vi "gauss on P&D.vi"(3 "error in (no error)":errorcluster, 4 "Coordinates":i32[](array[numeric]), 5 "click event":i32, 6 "gauss fit":bool) -> (0 "error out":errorcluster, 1 "fitted \ncoordinates":i32[](array[numeric]), 2 "Fit successful":bool)   [LabVIEW 2009]
uses:
  <vilib>/vision/NI_Vision_Development_Module.lvlib
panel:
  out "selection":T1(plugin-control)
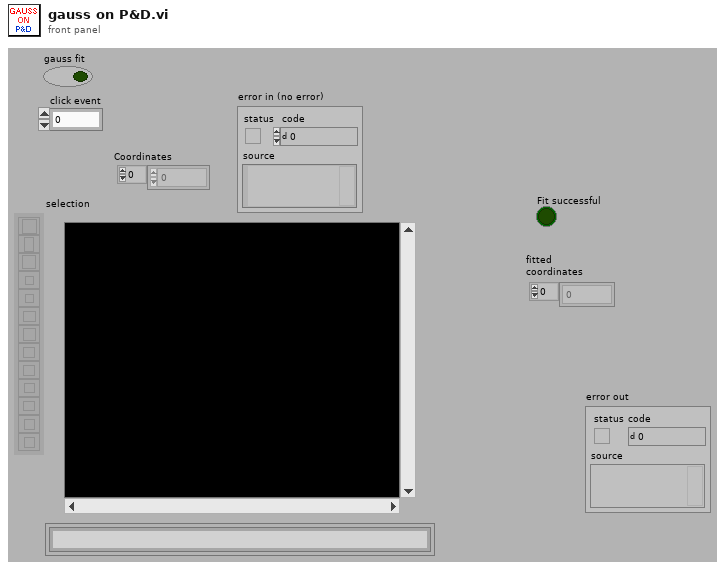
[diagram p1: front panel]
types:
  T1 = typedef "IMAQ Image.ctl" = refnum<image>
  T2 = typedef "DAQLinescanVisualization.ctt" = cluster{"Threshold":u32, "Trace Window #":u32, "IMAQ Trace":T1, "Retrace Window #":u32, "IMAQ Retrace":T1}
  T3 = typedef "Image Type" = u32
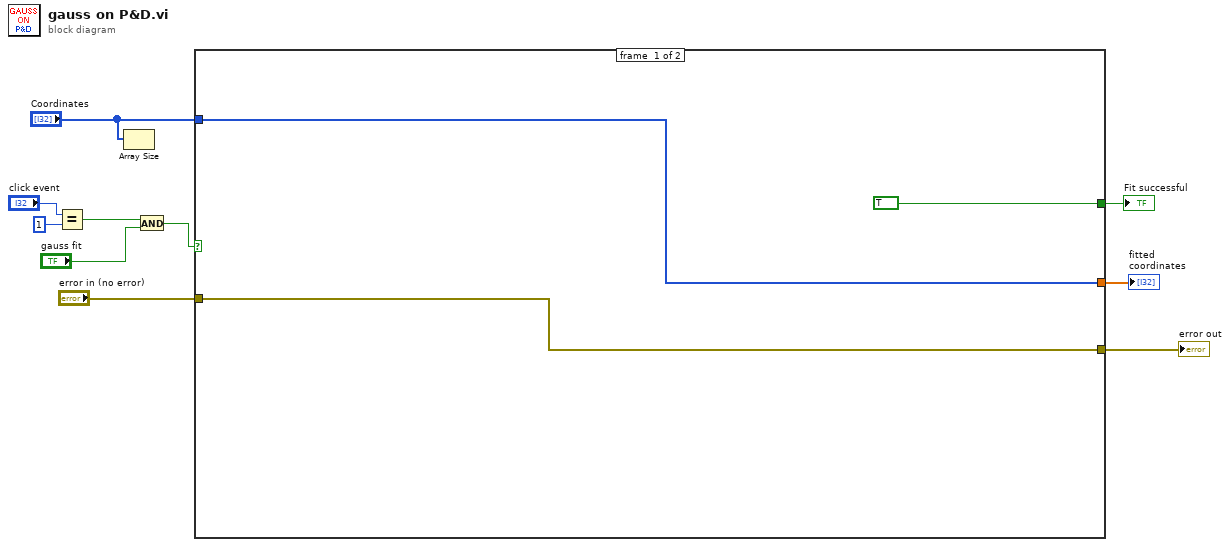
[diagram p0: block diagram]
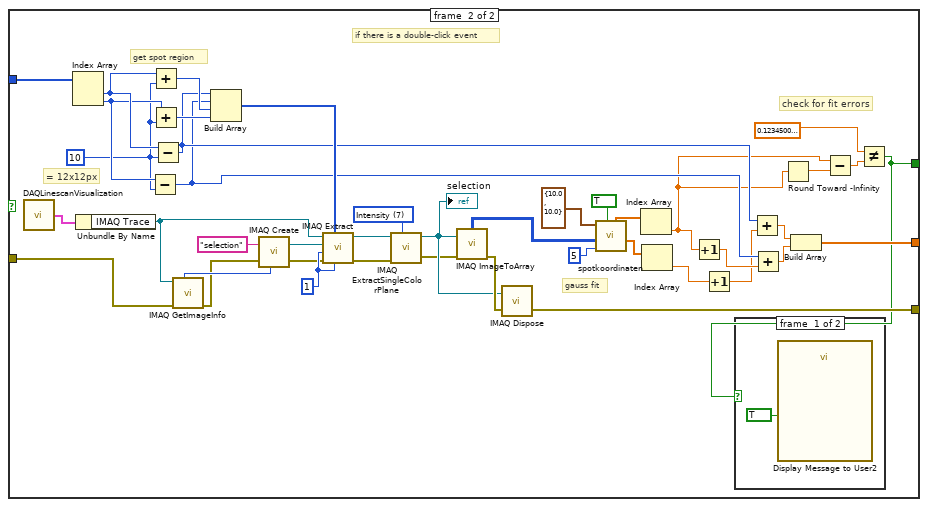
[diagram p2: hidden frame]
diagram:
  n1 = Equal?(x="click event", y=1) -> (x = y?=w2:bool)
  n2 = Array Size(array="Coordinates") -> ()  [unwired: 1 out]
  n3 = And(x=w2, y="gauss fit") -> (x .and. y?=w1:bool)
  n4 = case shown="True" w1 {
    tunnel: "Coordinates" -> [w12 w55]
    tunnel: "error in (no error)" -> [w13 w33]
    tunnel: [w13 w30] -> w8
    tunnel: [w12 w38] -> w7
    tunnel: [TRUE w29] -> w6
    frame #0 {
    }
    frame #1 {
      w24 = 7 items=["Red", "Green", "Blue", "Hue", "Saturation", "Luminance", "Value", "Intensity"] ("Color Plane")
      w51 = 10
      w52 = 1 ("X Step Size")
      # "check for fit errors"
      # "gauss fit"
      # "= 12x12px"
      # "get spot region"
      # "if there is a double-click event"
      n5 = call "DAQLinescanVisualization.vi"() -> ("Visualization (output)"=w27:T2)  [unwired: 2 in]
      n6 = Index Array(array=w55) -> (element #1=w54:i32, element #2=w53:i32)  [unwired: 2 in]
      n7 = Unbundle By Name(w27) -> ("IMAQ Trace"=w35:T1)
      n8 = Subtract(x=w53, y=w51) -> (x-y=w18:i32)
      n9 = Add(x=w54, y=w51) -> (x+y=w21:i32)
      n10 = Add(x=w53, y=w51) -> (x+y=w20:i32)
      n11 = Subtract(x=w54, y=w51) -> (x-y=w19:i32)
      n12 = call "IMAQ GetImageInfo"("error in (no error)"=w33, "Image"=w35) -> ("error out"=w32:errorcluster, "Image Type"=w34:T3)  [unwired: 2 in, 6 out]
      n13 = Build Array(w19, w18, w21, w20) -> (w50:i32[])
      n14 = call "IMAQ Create"("Image Name"="selection", "Image Type"=w34, "error in (no error)"=w32) -> ("New Image"=w42:T1, "error out"=w41:errorcluster)  [unwired: 2 in]
      n15 = call "IMAQ Extract"("Y Step Size"=w52, "Optional Rectangle"=w50, "error in (no error)"=w41, "X Step Size"=w52, "Image Dst"=w42, "Image Src"=w35) -> ("error out"=w23:errorcluster, "Image Dst Out"=w26:T1)  [unwired: 4 in]
      n16 = call "IMAQ ExtractSingleColorPlane"("Color Plane"=w24, "error in (no error)"=w23, "Image Src"=w26) -> ("error out"=w22:errorcluster, "Image Dst Out"=w25:T1)  [unwired: 7 in]
      "selection" <- w25
      n17 = call "IMAQ ImageToArray"("error in (no error)"=w22, "Image"=w25) -> ("error out"=w31:errorcluster, "Image Pixels (U8)"=w49:u8[][])  [unwired: 2 in, 3 out]
      n18 = call "IMAQ Dispose"("Image"=w25, "error in (no error)"=w31) -> ("error out"=w30:errorcluster)  [unwired: 4 in]
      n19 = call "spotkoordinaten.vi"("Gauss"=TRUE, "Area"=5, "Image"=w49, "Center of Mass"=cluster{"X":dbl, "Y":dbl} {"X"=10.0, "Y"=10.0}) -> ("yValues"=w44:dbl[], "xValues"=w45:dbl[])  [unwired: 1 in, 3 out]
      n20 = Index Array(array=w45) -> (element=w17:dbl)  [unwired: 1 in]
      n21 = Index Array(array=w44) -> (element=w15:dbl)  [unwired: 1 in]
      n22 = Increment(x=w17) -> (x+1=w16:dbl)
      n23 = Increment(x=w15) -> (x+1=w14:dbl)
      n24 = Add(x=w19, y=w14) -> (x+y=w40:dbl)
      n25 = Add(x=w18, y=w16) -> (x+y=w39:dbl)
      n26 = Round Toward -Infinity(1:w17) -> (0:w37:dbl)
      n27 = Build Array(w40, w39) -> (w38:dbl[])
      n28 = Subtract(x=w17, y=w37) -> (x-y=w36:dbl)
      n29 = Not Equal?(x=0.12345000000000006 ("x-y"), y=w36) -> (x != y?=w29:bool)
      n30 = case shown="False" w29 {
        frame #0 {
          n31 = call "Display Message to User2"("Enable"=TRUE) -> ()  [unwired: 9 in, 2 out]
        }
        frame #1 {
        }
      }
    }
  }
  "error out" <- w8
  "fitted \ncoordinates" <- w7
  "Fit successful" <- w6
